vi "connect To Cyclone.vi"(8 "error in":errorcluster, 11 "nameIpOrPortIdentifier":string) -> (0 "error out":errorcluster, 2 "function return":u32, 3 "nameIpOrPortIdentifier out":string)   [LabVIEW 2021, in "CycloneControlSDK.lvlib"]
doc: "extern \"C\" uint32_t _cdecl connectToCyclone(char *nameIpOrPortIdentifier);"
uses:
  CycloneControlSDK.lvlib
  CycloneControlSDK_64.dll
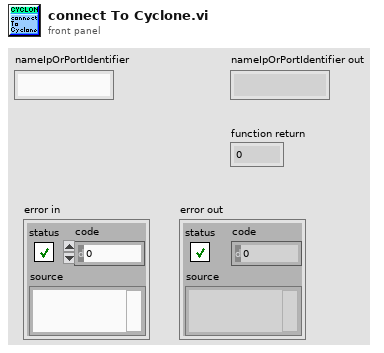
[diagram p1: front panel]
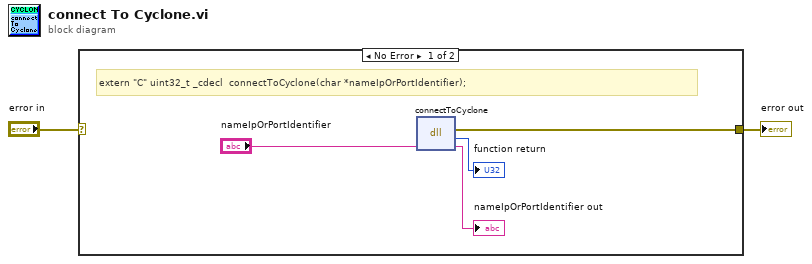
[diagram p0: block diagram]
diagram:
  n1 = case shown="No Error" "error in" {
    selector: "error in" -> [_ w7]
    tunnel: [w3 w7] -> w1
    frame No Error {
      # "extern \"C\" uint32_t _cdecl  connectToCyclone(char *nameIpOrPortIdentifier);"
      n2 = dll-call lib="C:/PEMicro/cyclone/cycloneControl/controlsdk/examples/labview2018/user.lib/CycloneControlSDK/CycloneControlSDK_64.dll" fn="connectToCyclone"("nameIpOrPortIdentifier"="nameIpOrPortIdentifier") -> (error out=w3:errorcluster, "return type"=→"function return":u32, "nameIpOrPortIdentifier"=→"nameIpOrPortIdentifier out":string)  [unwired: 3 in, 1 out]
    }
    frame Error {
    }
  }
  "error out" <- w1
